vi "_Subscribe.vi"(4 "IP Resolver":refnum<class "IP Resolver.lvclass">, 6 "EventLogging":refnum<class "EventLoggingService.lvclass">, 8 "error in (no error)":errorcluster, 9 "DataHandler":refnum<class "SubscribedDataHandler.lvclass">, 10 "Subscription":T1, 11 "Loop Data In":T2) -> (0 "error out":errorcluster, 3 "Loop Data":T2)   [LabVIEW 2020, in "Vecto.lvlib" / "RemoteDataService.lvclass"]
uses:
  RemoteDataService.lvclass
  Loop Data.ctl
  SequenceCountService/SequenceCountService.lvclass
  ChannelService/ChannelService.lvclass
  Published Group.ctl
  Packet.ctl
  lv-protoc/LV-Proto/Message/Message.lvclass
  Group Data Type.ctl
  Subscription.ctl
  Subscription Info.ctl
  SubscribedDataHandler/SubscribedDataHandler.lvclass
  VectoConfig/Telemetry Config.ctl
  VectoConfig/Telemetry Routing.ctl
  VectoConfig/Endpoint.ctl
  EventLoggingService/EventLoggingService.lvclass
  IP Resolver/IP Resolver.lvclass
  Event Level.ctl
  EventLoggingService/EventLoggingService.lvclass/EventLoggingService.ctl
  <vilib>/Utility/error.llb/Error Cluster From Error Code.vi
  EventLogHandler/EventLogHandler.lvclass
  RemoteDataService.lvclass/RemoteDataService.ctl
  TCPMessaging/TCPMessaging.lvclass
  Vecto.lvlib
  VectoConfig/VectoConfig.lvlib
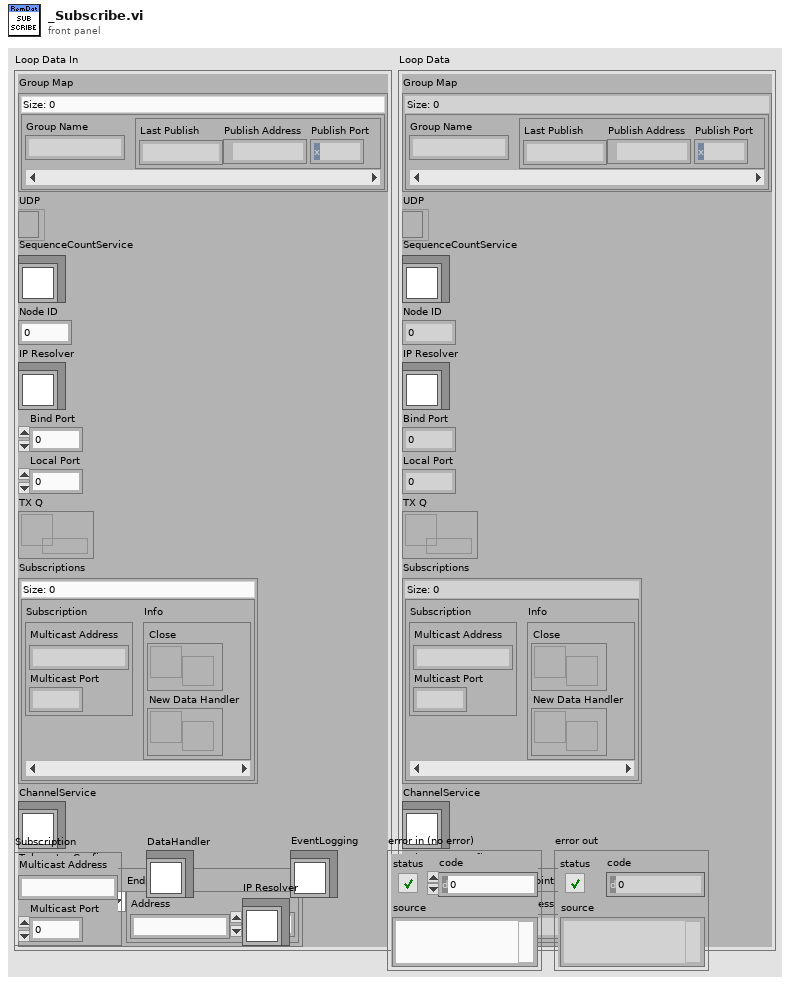
[diagram p1: front panel]
types:
  T1 = typedef "Vecto.lvlib/RemoteDataService.lvclass/Subscription.ctl" = cluster{"Multicast Address":string, "Multicast Port":u16}
  T2 = typedef "Vecto.lvlib/RemoteDataService.lvclass/Loop Data.ctl" = cluster{"Group Map":map{string, T3}, "UDP":refnum<k16>, "SequenceCountService":refnum<class "SequenceCountService.lvclass">, "Node ID":u32, "IP Resolver":refnum<class "IP Resolver.lvclass">, "Bind Port":u16, "Local Port":u16, "TX Q":refnum<queue>, "Subscriptions":map{T1, T4}, "ChannelService":refnum<class "ChannelService.lvclass">, "Telemetry Config":T5}
  T3 = typedef "Vecto.lvlib/RemoteDataService.lvclass/Published Group.ctl" = cluster{"Last Publish":dbl, "Publish Address":u32, "Publish Port":u16}
  T4 = typedef "Vecto.lvlib/RemoteDataService.lvclass/Subscription Info.ctl" = cluster{"Close":refnum<user-event>, "New Data Handler":refnum<user-event>}
  T5 = typedef "VectoConfig.lvlib/Telemetry Config.ctl" = cluster{"Routing":T6, "Endpoint":T7}
  T6 = typedef "VectoConfig.lvlib/Telemetry Routing.ctl" = enum16{"Multicast", "Unicast"}
  T7 = typedef "VectoConfig.lvlib/Endpoint.ctl" = cluster{"Address":string, "Port":u16}
  T8 = typedef "Vecto.lvlib/Event Level.ctl" = enum16{"Debug", "Info", "Warning", "Error"}
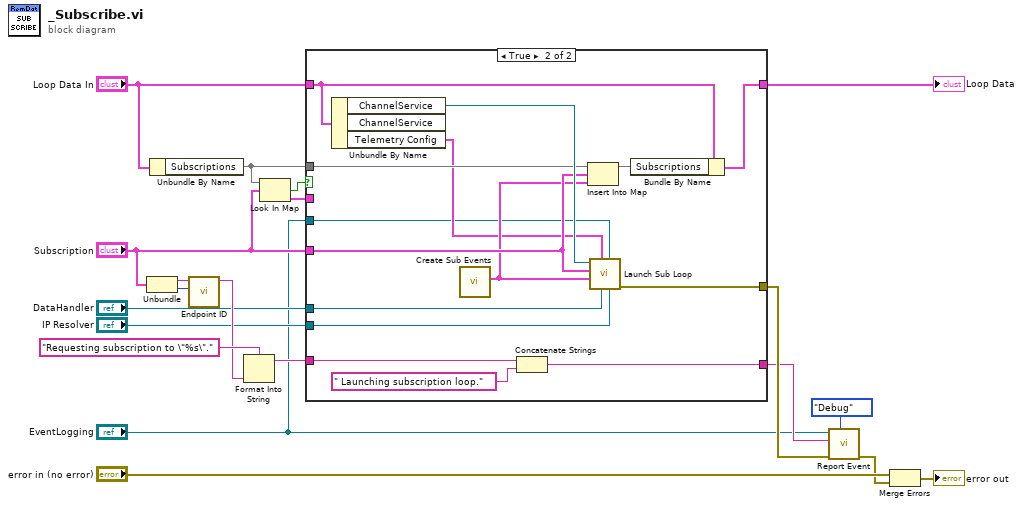
[diagram p0: block diagram]
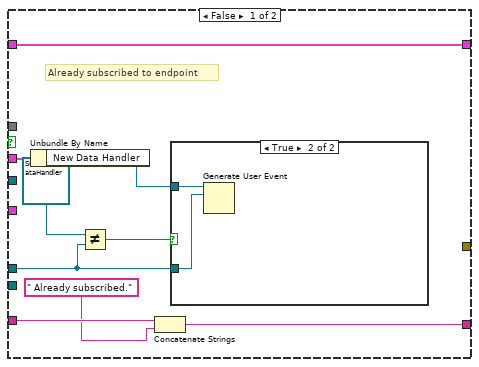
[diagram p2: hidden frame]
diagram:
  n1 = Unbundle("Subscription") -> ("Multicast Address"=w11:string, "Multicast Port"=w10:u16)
  n2 = Unbundle By Name("Loop Data In") -> ("Subscriptions"=w18:map{T1, T4})
  n3 = call "Endpoint ID.vi"("Remote Port"=w10, "Remote Address"=w11) -> ("Endpoint ID"=w8:string)  [unwired: 9 in]
  n4 = Format Into String(format string="Requesting subscription to \"%s\".", w8) -> (resulting string=w7:string)  [unwired: 2 in, 1 out]
  n5 = Look In Map(map=w18, key="Subscription") -> (key not found?=w19:bool, value=w17:T4)  [unwired: 1 in]
  n6 = case shown="True" w19 {
    tunnel: w18 -> [_ w45]
    tunnel: w17 -> [w23 _]
    tunnel: "Subscription" -> [_ w44]
    tunnel: "Loop Data In" -> [w29 w43]
    tunnel: [w29 w41] -> w14
    tunnel: [_ w40] -> w20
    tunnel: w7 -> [w28 w39]
    tunnel: [w26 w37] -> w4
    tunnel: "DataHandler" -> [w22 w35]
    tunnel: "IP Resolver" -> [_ w34]
    tunnel: "EventLogging" -> [_ w32]
    frame False {
      # "Already subscribed to endpoint"
      n7 = Unbundle By Name(w23) -> ("New Data Handler"=w21:refnum<user-event>)
      n8 = Not Equal?(x=refnum<class "SubscribedDataHandler.lvclass"> refnum, y=w22) -> (x != y?=w24:bool)
      n9 = Concatenate Strings(w28, " Already subscribed.") -> (w26:string)
      n10 = case shown="True" w24 {
        tunnel: w22 -> [_ w30]
        tunnel: w21 -> [_ w31]
        frame False {
        }
        frame True {
          n11 = Generate User Event(user event=w31, event data cluster=w30) -> ()  [unwired: 2 in, 2 out]
        }
      }
    }
    frame True {
      n12 = Unbundle By Name(w43) -> ("ChannelService"=w46:refnum<class "ChannelService.lvclass">, "Telemetry Config"=w33:T5)  [unwired: 1 out]
      n13 = call "Create Sub Events.vi"() -> ("Sub Events"=w36:T4)  [unwired: 11 in]
      n14 = Concatenate Strings(w39, " Launching subscription loop.") -> (w37:string)
      n15 = Insert Into Map(map in=w45, key=w44, value=w36) -> (map out=w42:map{T1, T4})  [unwired: 2 out]
      n16 = call "Launch Sub Loop.vi"("IP Resolver"=w34, "EventLogging"=w32, "DataHandler"=w35, "Telemetry Config"=w33, "Subscription Info"=w36, "Subscription"=w44, "ChannelService"=w46) -> ("error out"=w40:errorcluster)  [unwired: 4 in]
      n17 = Bundle By Name(cluster=w43, "Subscriptions"=w42) -> (w41:T2)
    }
  }
  "Loop Data" <- w14
  n18 = call "Report Event.vi"("Event Level (Info)"=Event_Level."Debug", "error in (no error)"=w20, "Message"=w4, "EventLoggingService in"="EventLogging") -> ("error out"=w5:errorcluster)  [unwired: 6 in, 1 out]
  n19 = Merge Errors("error in (no error)", w5) -> (→"error out":errorcluster)
